vi "4_7.vi"() -> ()   [LabVIEW 2015]
panel:
  in  "Error In":errorcluster
  in  "Stop Button":bool
  out "Waveform Graph":dynamicdata(graph)
  in  "Duty Cycle":dbl
  in  "Phase":dbl
  in  "Amplitude [V]":dbl
  in  "Offset [V]":dbl
  in  "Reset Signal":bool
  in  "Frequency [Hz]":dbl(knob) scale=0.0..1000.0
  in  "Enum":T1(ring)
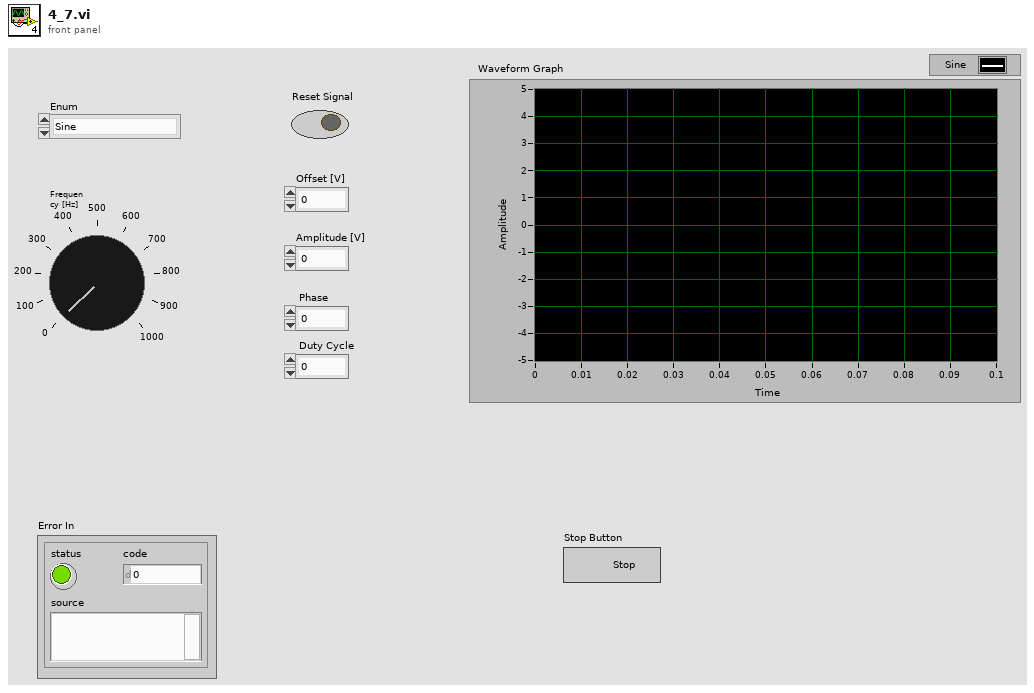
[diagram p1: front panel]
types:
  T1 = enum16{"Sine", "Square", "Triangle", "Sawtooth", "DC", ""}
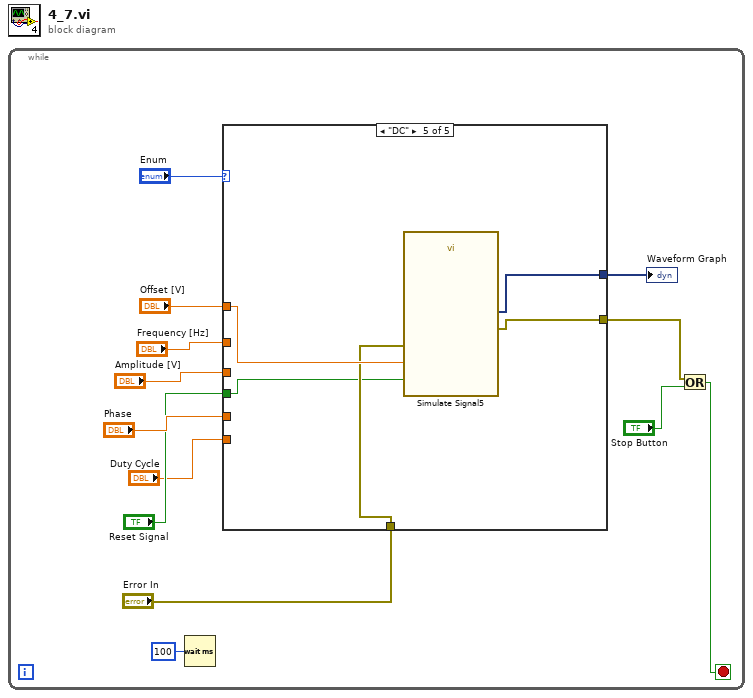
[diagram p0: block diagram]
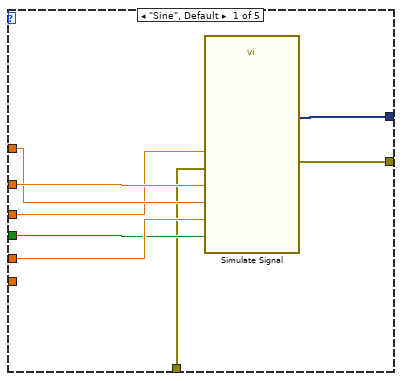
[diagram p2: hidden frame]
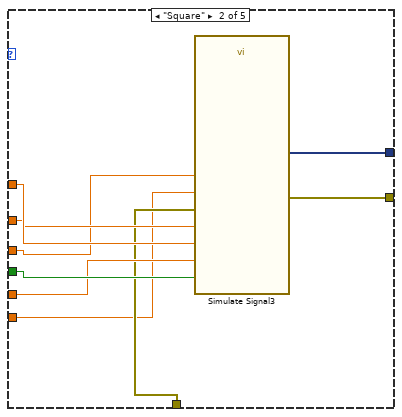
[diagram p3: hidden frame]
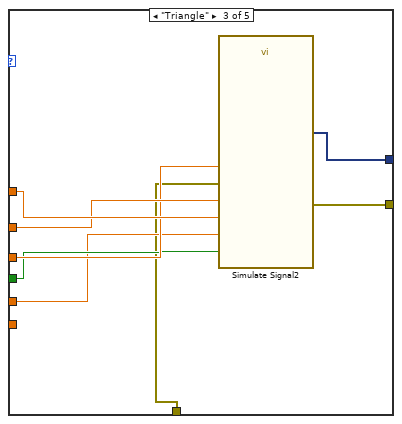
[diagram p4: hidden frame]
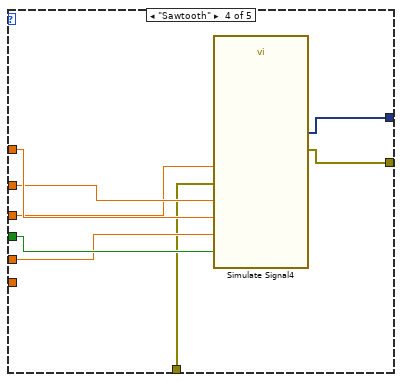
[diagram p5: hidden frame]
diagram:
  n1 = while {
    stop <- w3 stop-if-true
    n2 = Wait (ms)(milliseconds to wait=u32 100) -> ()  [unwired: 1 out]
    n3 = case shown="\"DC\"" "Enum" {
      tunnel: [w21 w23 w32 w39 w47] -> w12
      tunnel: "Offset [V]" -> [w19 w30 w38 w46 w51]
      tunnel: "Frequency [Hz]" -> [w20 w29 w37 w45 _]
      tunnel: "Amplitude [V]" -> [w18 w28 w36 w44 _]
      tunnel: "Phase" -> [w17 w26 w34 w42 _]
      tunnel: "Reset Signal" -> [w16 w27 w35 w43 w49]
      tunnel: "Duty Cycle" -> [_ w22 _ _ _]
      tunnel: [w15 w24 w33 w40 w48] -> w5
      tunnel: "Error In" -> [w14 w25 w31 w41 w50]
      frame "Sine", Default {
        n4 = call "Simulate Signal"("Offset"=w19, "Reset Signal"=w16, "Frequency"=w20, "Amplitude"=w18, "Phase"=w17, "error in (no error)"=w14) -> ("Sine"=w21:dynamicdata, "error out"=w15:errorcluster)  [unwired: 8 in]
      }
      frame "Square" {
        n5 = call "Simulate Signal3"("Offset"=w30, "Duty Cycle (%)"=w22, "Reset Signal"=w27, "Frequency"=w29, "Amplitude"=w28, "Phase"=w26, "error in (no error)"=w25) -> ("Square"=w23:dynamicdata, "error out"=w24:errorcluster)  [unwired: 7 in]
      }
      frame "Triangle" {
        n6 = call "Simulate Signal2"("Offset"=w38, "Reset Signal"=w35, "Frequency"=w37, "Amplitude"=w36, "Phase"=w34, "error in (no error)"=w31) -> ("Triangle"=w32:dynamicdata, "error out"=w33:errorcluster)  [unwired: 8 in]
      }
      frame "Sawtooth" {
        n7 = call "Simulate Signal4"("Offset"=w46, "Reset Signal"=w43, "Frequency"=w45, "Amplitude"=w44, "Phase"=w42, "error in (no error)"=w41) -> ("Sawtooth"=w39:dynamicdata, "error out"=w40:errorcluster)  [unwired: 8 in]
      }
      frame "DC" {
        n8 = call "Simulate Signal5"("Offset"=w51, "Reset Signal"=w49, "error in (no error)"=w50) -> ("DC"=w47:dynamicdata, "error out"=w48:errorcluster)  [unwired: 11 in]
      }
    }
    "Waveform Graph" <- w12
    n9 = Or(x=w5, y="Stop Button") -> (x .or. y?=w3:bool)
  }
